vi "distanceFormula.vi"(8 "Y2":dbl, 9 "X2":dbl, 10 "Y1":dbl, 11 "X1":dbl) -> (3 "Distance":dbl)   [LabVIEW 2011]
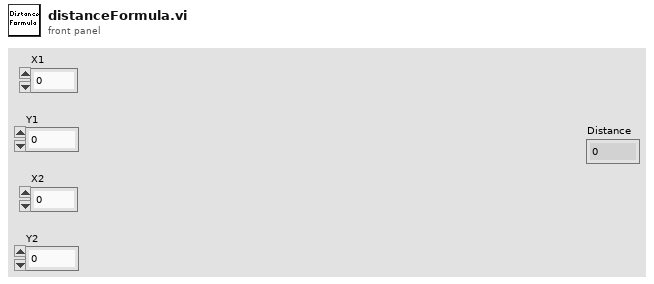
[diagram p1: front panel]
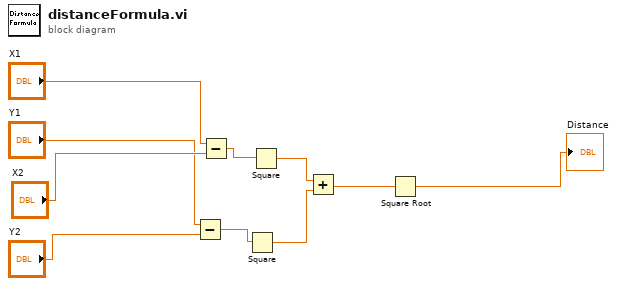
[diagram p0: block diagram]
diagram:
  n1 = Subtract(x="Y1", y="Y2") -> (x-y=w5:dbl)
  n2 = Subtract(x="X1", y="X2") -> (x-y=w6:dbl)
  n3 = Square(x=w5) -> (x^2=w4:dbl)
  n4 = Square(x=w6) -> (x^2=w3:dbl)
  n5 = Add(x=w3, y=w4) -> (x+y=w2:dbl)
  n6 = Square Root(x=w2) -> (sqrt(x)=→"Distance":dbl)
